vi "Manual panel.vi"() -> ()   [LabVIEW 2016]
panel:
  in  "OFF":bool
  in  "STD":bool
  in  "ABN":bool
  in  "FLT":bool
  in  "FLT":bool
  in  "ABN":bool
  in  "BKS":bool
  in  "I2G":bool
  in  "STD":bool
  in  "G2I_IN":bool
  in  "G2I_UN":bool
  in  "ISD":bool
  in  "GC":bool
  in  "ISD":bool
  in  "FLT":bool
  in  "ABN":bool
  in  "BKS":bool
  in  "STD":bool
  in  "GC":bool
  in  "FLT":bool
  in  "ABN":bool
  in  "I2G":bool
  in  "STD":bool
  in  "G2I_IN":bool
  in  "FLT":bool
  in  "ABN":bool
  in  "ISD":bool
  in  "STD":bool
  in  "G2I_UN":bool
  in  "FLT":bool
  in  "ABN":bool
  in  "ISD":bool
  in  "STD":bool
  in  "FLT":bool
  in  "ABN":bool
  in  "ISD":bool
  in  "I2G":bool
  in  "FLT":bool
  in  "ABN":bool
  in  "G2I_IN":bool
  in  "G2I_UN":bool
  in  "GC":bool
  in  "FLT":bool
  in  "ABN":bool
  in  "STD":bool
  in  "BKS":bool
  in  "ISD":bool
  in  "GC":bool
  in  "STD":bool
  in  "ABN":bool
  in  "FLT":bool
  # "OFF State"
  # "STD State"
  # "GC State"
  # "BKS State"
  # "ISD State"
  # "ABN State"
  # "G2I_UN State"
  # "G2I_IN State"
  # "FLT State"
  # "I2G State"
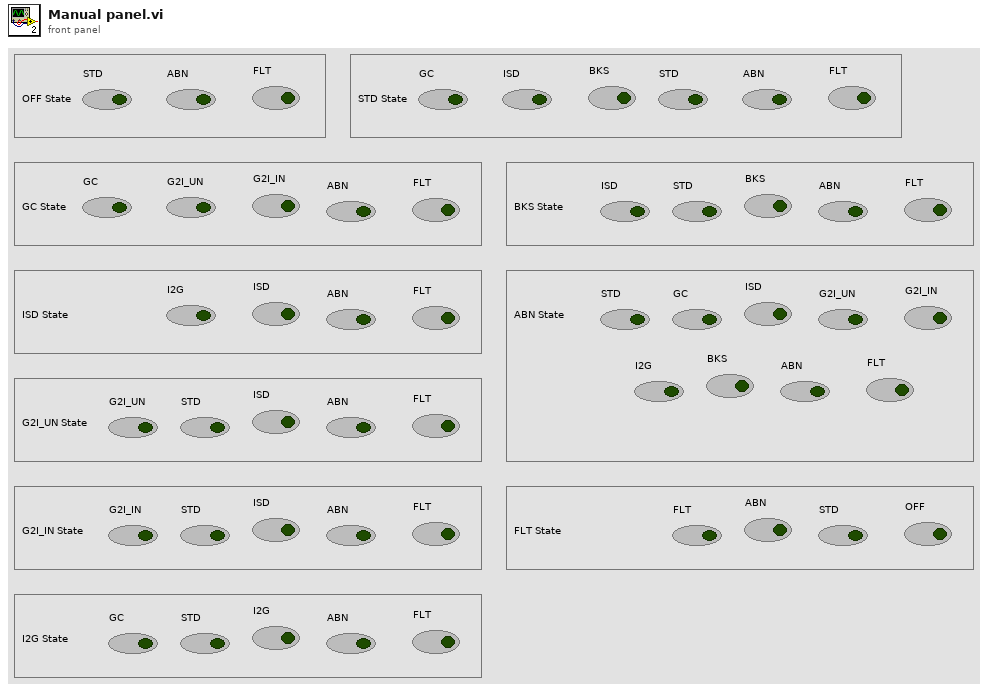
[diagram p1: front panel]
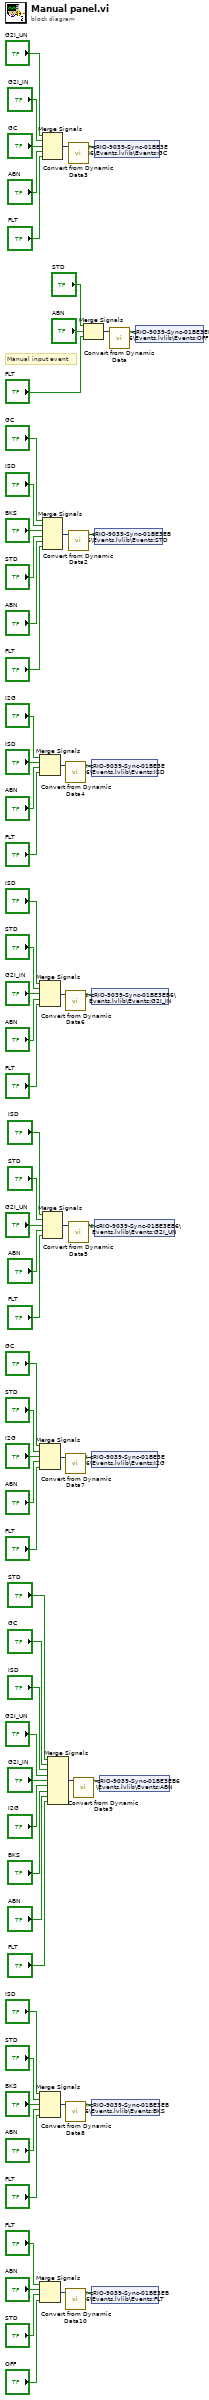
[diagram p0: block diagram]
diagram:
  # "Manual input event"
  n1 = Merge Signals("I2G", "ISD", "ABN", "FLT") -> (w51:dynamicdata)
  n2 = Merge Signals("ISD", "STD", "G2I_IN", "ABN", "FLT") -> (w38:dynamicdata)
  n3 = Merge Signals("GC", "STD", "I2G", "ABN", "FLT") -> (w31:dynamicdata)
  n4 = Merge Signals("ISD", "STD", "BKS", "ABN", "FLT") -> (w24:dynamicdata)
  n5 = Merge Signals("FLT", "ABN", "STD", "OFF") -> (w6:dynamicdata)
  n6 = Merge Signals("G2I_UN", "G2I_IN", "GC", "ABN", "FLT") -> (w58:dynamicdata)
  n7 = Merge Signals("GC", "ISD", "BKS", "STD", "ABN", "FLT") -> (w66:dynamicdata)
  n8 = Merge Signals("ISD", "STD", "G2I_UN", "ABN", "FLT") -> (w45:dynamicdata)
  n9 = Merge Signals("STD", "GC", "ISD", "G2I_UN", "G2I_IN", "I2G", "BKS", "ABN", "FLT") -> (w17:dynamicdata)
  n10 = call "Convert from Dynamic Data4"("Dynamic Data Type"=w51) -> ("Array"=w50:bool[])  [unwired: 3 in]
  n11 = call "Convert from Dynamic Data6"("Dynamic Data Type"=w38) -> ("Array"=w37:bool[])  [unwired: 3 in]
  n12 = call "Convert from Dynamic Data7"("Dynamic Data Type"=w31) -> ("Array"=w30:bool[])  [unwired: 3 in]
  n13 = call "Convert from Dynamic Data8"("Dynamic Data Type"=w24) -> ("Array"=w23:bool[])  [unwired: 3 in]
  n14 = call "Convert from Dynamic Data10"("Dynamic Data Type"=w6) -> ("Array"=w5:bool[])  [unwired: 3 in]
  n15 = call "Convert from Dynamic Data3"("Dynamic Data Type"=w58) -> ("Array"=w57:bool[])  [unwired: 3 in]
  n16 = call "Convert from Dynamic Data2"("Dynamic Data Type"=w66) -> ("Array"=w65:bool[])  [unwired: 3 in]
  n17 = call "Convert from Dynamic Data5"("Dynamic Data Type"=w45) -> ("Array"=w44:bool[])  [unwired: 3 in]
  n18 = call "Convert from Dynamic Data9"("Dynamic Data Type"=w17) -> ("Array"=w16:bool[])  [unwired: 3 in]
  n19 = Merge Signals("STD", "ABN", "FLT") -> (w71:dynamicdata)
  n20 = shared-variable "NI-cRIO-9039-Sync-01BE3EB6\\Events.lvlib\\Events:ISD"(w50) -> ()  [unwired: 1 in, 1 out]
  n21 = shared-variable "NI-cRIO-9039-Sync-01BE3EB6\\Events.lvlib\\Events:G2I_IN"(w37) -> ()  [unwired: 1 in, 1 out]
  n22 = shared-variable "NI-cRIO-9039-Sync-01BE3EB6\\Events.lvlib\\Events:I2G"(w30) -> ()  [unwired: 1 in, 1 out]
  n23 = shared-variable "NI-cRIO-9039-Sync-01BE3EB6\\Events.lvlib\\Events:BKS"(w23) -> ()  [unwired: 1 in, 1 out]
  n24 = shared-variable "NI-cRIO-9039-Sync-01BE3EB6\\Events.lvlib\\Events:FLT"(w5) -> ()  [unwired: 1 in, 1 out]
  n25 = shared-variable "NI-cRIO-9039-Sync-01BE3EB6\\Events.lvlib\\Events:GC"(w57) -> ()  [unwired: 1 in, 1 out]
  n26 = shared-variable "NI-cRIO-9039-Sync-01BE3EB6\\Events.lvlib\\Events:STD"(w65) -> ()  [unwired: 1 in, 1 out]
  n27 = shared-variable "NI-cRIO-9039-Sync-01BE3EB6\\Events.lvlib\\Events:G2I_UN"(w44) -> ()  [unwired: 1 in, 1 out]
  n28 = shared-variable "NI-cRIO-9039-Sync-01BE3EB6\\Events.lvlib\\Events:ABN"(w16) -> ()  [unwired: 1 in, 1 out]
  n29 = call "Convert from Dynamic Data"("Dynamic Data Type"=w71) -> ("Array"=w70:bool[])  [unwired: 3 in]
  n30 = shared-variable "NI-cRIO-9039-Sync-01BE3EB6\\Events.lvlib\\Events:OFF"(w70) -> ()  [unwired: 1 in, 1 out]
